vi "Calculate FPS.vi"(7 "Frames Processed":dbl=1.0) -> (2 "Fps":dbl)   [LabVIEW 2019]
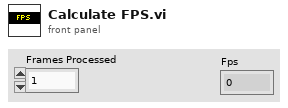
[diagram p1: front panel]
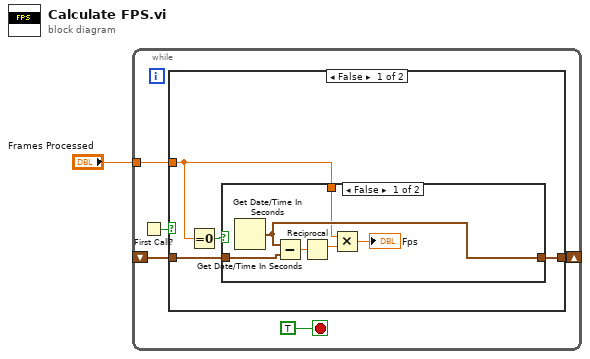
[diagram p0: block diagram]
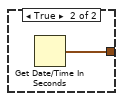
[diagram p3: hidden frame]
diagram:
  n1 = while {
    shift-right: [w5] -> _
    shift-left: _ -> [w6]
    tunnel: "Frames Processed" -> [w2]
    stop <- TRUE stop-if-true
    n2 = First Call?() -> (First Call?: T/F=w3:bool)
    n3 = case shown="False" w3 {
      tunnel: w6 -> [w10 _]
      tunnel: [w9 w18] -> w5
      tunnel: w2 -> [w8 _]
      frame False {
        n4 = Equal To 0?(x=w8) -> (x = 0?=w7:bool)
        n5 = case shown="False" w7 {
          tunnel: w10 -> [w16 w17]
          tunnel: [w15 w17] -> w9
          tunnel: w8 -> [w12 _]
          frame False {
            n6 = Get Date/Time In Seconds() -> ()  [unwired: 1 out]
            n7 = Get Date/Time In Seconds() -> (seconds since 1Jan1904=w15:timestamp)
            n8 = Subtract(x=w15, y=w16) -> (x-y=w14:dbl)
            n9 = Reciprocal(x=w14) -> (1/x=w13:dbl)
            n10 = Multiply(x=w12, y=w13) -> (x*y=→"Fps":dbl)
          }
          frame True {
          }
        }
      }
      frame True {
        n11 = Get Date/Time In Seconds() -> (seconds since 1Jan1904=w18:timestamp)
      }
    }
  }
